vi "Demo - Continuous Capture.vi"() -> ()   [LabVIEW 2017]
uses:
  Communications/Typedefs/Data Size--Enum.ctl
  Communications/Communications Library.lvlib
  GUI/Consoles/Communications Console Library.lvlib
panel:
  in  "Data Size":T1
  in  "Show Console":bool
  in  "configuration file path":path
  out "Capture Rate (Bytes/Second)":dbl format="%#_4p"
  out "Waveform Graph":i32[][](graph)
  in  "stop":bool
  in  "Buffer Block Size (Samples per channel)":i32=256
  out "error out":errorcluster
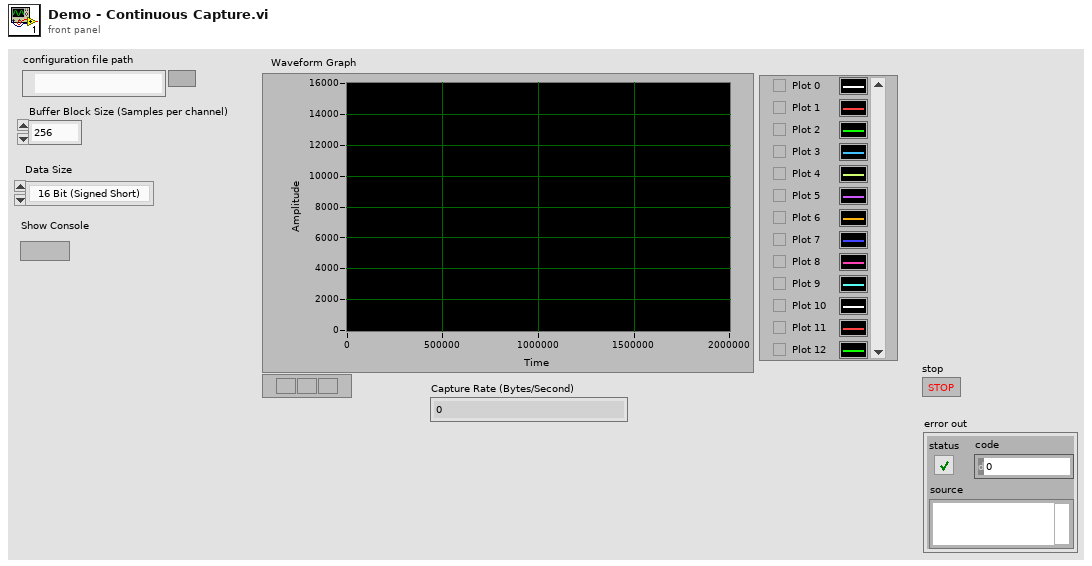
[diagram p1: front panel]
types:
  T1 = typedef "Communications Library.lvlib/Data Size--Enum.ctl" = enum16{"16 Bit (Signed Short)", "32 Bit (Signed Long)"}
  T2 = typedef "Communications Library.lvlib/DTACQ Module Carrier Configuration--Cluster.ctl" = cluster{"Name":string, "IP":string, "Control Port":i32, "Timeout (ms)":i32, "Continuous Capture Port (Multiplexed)":i32, "Start HIL Shot Port":i32, "AWG Upload Port (Multiplexed)":i32, "Download Captured Data Port (Multiplexed)":i32, "Module Slots":i32, "Module Configurations":T3[]}
  T3 = typedef "Communications Library.lvlib/DTACQ Module Configuration--Cluster.ctl" = cluster{"Name":string, "Position":string, "Module Type":T4, "Control Port":i32, "Timeout (ms)":i32, "Channels":i32}
  T4 = typedef "Communications Library.lvlib/DTACQ Device Type--Enum.ctl" = enum16{"Carrier", "Analog In Module", "Analog Out Module", "Generic Module"}
  T5 = typedef "Communications Library.lvlib/DTACQ Connection Data--Cluster.ctl" = cluster{"Description":string, "Address":string, "Port":u16, "timeout (ms)":i32, "Termination Character":string, "TCP Connection Reference":refnum<k5>, "Open Connection":bool}
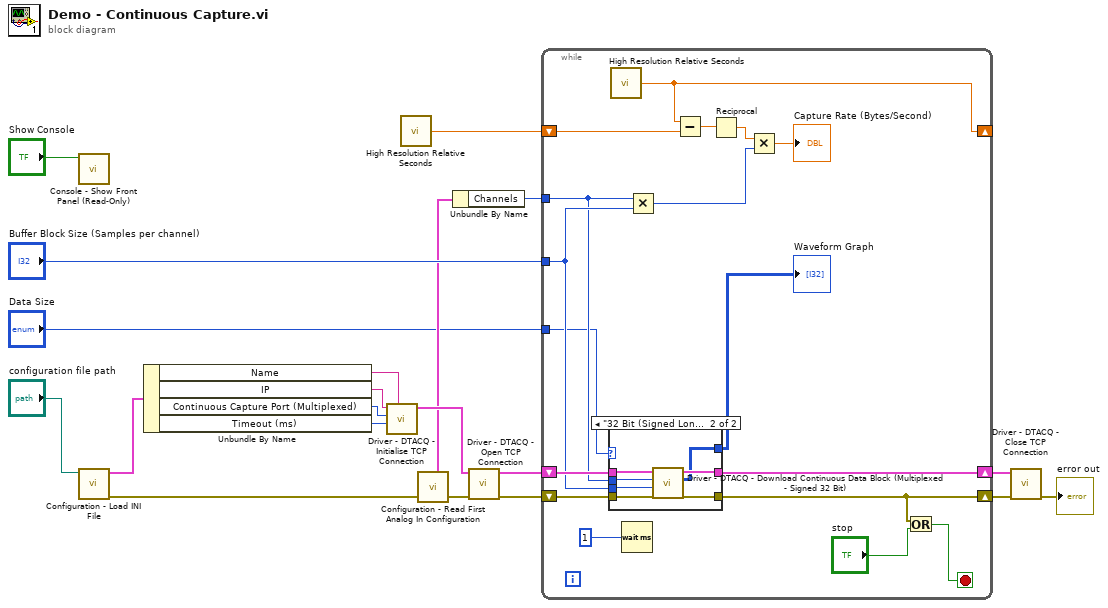
[diagram p0: block diagram]
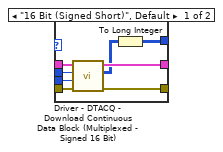
[diagram p2: hidden frame]
diagram:
  n1 = call "Console - Show Front Panel (Read-Only).vi"("Display Console"="Show Console") -> ()  [unwired: 11 in]
  n2 = call "Configuration - Load INI File.vi"("configuration file path"="configuration file path") -> ("error out"=w5:errorcluster, "Carrier Configuration Out"=w13:T2)  [unwired: 9 in]
  n3 = Unbundle By Name(w13) -> ("Name"=w12:string, "IP"=w11:string, "Continuous Capture Port (Multiplexed)"=w10:i32, "Timeout (ms)"=w9:i32)
  n4 = call "Driver - DTACQ - Initialise TCP Connection.vi"("Description"=w12, "timeout (ms)"=w9, "Port"=w10, "Address"=w11) -> ("DTACQ Connection Data Out"=w18:T5)  [unwired: 7 in]
  n5 = call <vilib>:"High Resolution Relative Seconds.vi"() -> ("relative seconds"=w16:dbl)
  n6 = call "Configuration - Read First Analog In Configuration.vi"("error in"=w5) -> ("error out"=w6:errorcluster, "AI - Module Configuration"=w4:T3)  [unwired: 6 in, 3 out]
  n7 = Unbundle By Name(w4) -> ("Channels"=w3:i32)
  n8 = call "Driver - DTACQ - Open TCP Connection.vi"("error in"=w6, "DTACQ Connection Data In"=w18) -> ("error out"=w8:errorcluster, "DTACQ Connection Data Out"=w7:T5)  [unwired: 8 in]
  n9 = while {
    shift-right: [w24] -> w20
    shift-left: w8 -> [w37]
    tunnel: w3 -> [w26]
    tunnel: "Buffer Block Size (Samples per channel)" -> [w27]
    shift-right: [w35] -> w17
    shift-left: w7 -> [w36]
    shift-right: [w28] -> _
    shift-left: w16 -> [w29]
    tunnel: "Data Size" -> [w21]
    stop <- w22 stop-if-true
    n10 = case shown="\"32 Bit (Signed Long)\"" w21 {
      tunnel: w37 -> [w45 w52]
      tunnel: w36 -> [w44 w51]
      tunnel: [w43 w48] -> w35
      tunnel: [w39 w46] -> w30
      tunnel: w27 -> [w42 w49]
      tunnel: w26 -> [w41 w50]
      tunnel: [w40 w47] -> w24
      frame "16 Bit (Signed Short)", Default {
        n11 = call "Driver - DTACQ - Download Continuous Data Block (Multiplexed - Signed 16 Bit).vi"("error in"=w45, "Number of Samples"=w42, "Number of Channels"=w41, "DTACQ Connection Data In"=w44) -> ("error out"=w40:errorcluster, "Data"=w38:i16[][], "DTACQ Connection Data Out"=w43:T5)  [unwired: 4 in, 1 out]
        n12 = To Long Integer(number=w38) -> (32bit integer=w39:i32[][])
      }
      frame "32 Bit (Signed Long)" {
        n13 = call "Driver - DTACQ - Download Continuous Data Block (Multiplexed - Signed 32 Bit).vi"("error in"=w52, "Number of Samples"=w49, "Number of Channels"=w50, "DTACQ Connection Data In"=w51) -> ("error out"=w47:errorcluster, "Data"=w46:i32[][], "DTACQ Connection Data Out"=w48:T5)  [unwired: 4 in, 1 out]
      }
    }
    "Waveform Graph" <- w30
    n14 = call <vilib>:"High Resolution Relative Seconds.vi"() -> ("relative seconds"=w28:dbl)
    n15 = Wait (ms)(milliseconds to wait=u32 1) -> ()  [unwired: 1 out]
    n16 = Multiply(x=w26, y=w27) -> (x*y=w25:i32)
    n17 = Subtract(x=w28, y=w29) -> (x-y=w33:dbl)
    n18 = Reciprocal(x=w33) -> (1/x=w32:dbl)
    n19 = Multiply(x=w32, y=w25) -> (x*y=→"Capture Rate (Bytes/Second)":dbl)
    n20 = Or(x=w24, y="stop") -> (x .or. y?=w22:bool)
  }
  n21 = call "Driver - DTACQ - Close TCP Connection.vi"("error in"=w20, "DTACQ Connection Data In"=w17) -> ("error out"=→"error out":errorcluster)  [unwired: 8 in, 1 out]
